vi "Read Period in ms.vi"(8 "error in (no error)":errorcluster, 11 "Poll Msg in":refnum<class "Poll Msg.lvclass">) -> (0 "error out":errorcluster, 2 "Period in ms":u32, 3 "Poll Msg out":refnum<class "Poll Msg.lvclass">)   [LabVIEW 2024, in "Poll Msg.lvclass"]
uses:
  Poll Msg.lvclass
  Poll Msg.lvclass/Poll Msg.ctl
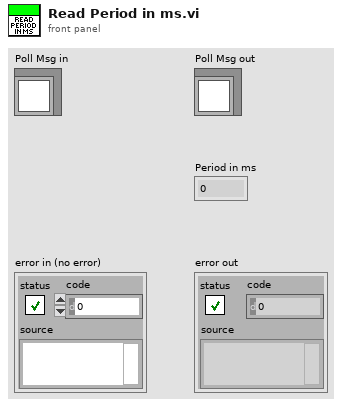
[diagram p1: front panel]
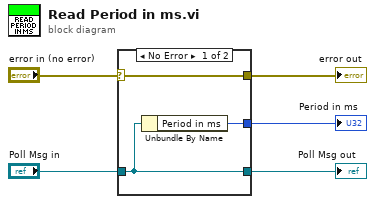
[diagram p0: block diagram]
diagram:
  n1 = case shown="No Error" "error in (no error)" {
    selector: "error in (no error)" -> [w8 w9]
    tunnel: [w8 w9] -> w4
    tunnel: [w7 w10] -> w2
    tunnel: "Poll Msg in" -> [w7 w10]
    tunnel: [w6 _] -> w1
    frame No Error {
      n2 = Unbundle By Name(w7) -> ("Period in ms"=w6:u32)
    }
    frame Error {
    }
  }
  "error out" <- w4
  "Poll Msg out" <- w2
  "Period in ms" <- w1
